vi "close camera.vi"(8 "error in (no error)":errorcluster, 11 "Camera":T1) -> (0 "error out":errorcluster, 3 "Camera out":T1)   [LabVIEW 2022 SP3, in "Vision.lvlib"]
uses:
  Vision.lvlib
  camera.ctl
  camera driver.ctl
  C:/Users/Caleb/Desktop/nebraska-silicon-lab/pixel-gantry-extra/LV/bin/uEyeDotNet.dll
  bin/uEyeDotNet.dll
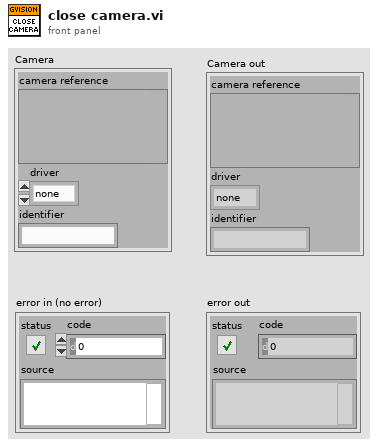
[diagram p1: front panel]
types:
  T1 = typedef "Vision.lvlib/camera.ctl" = cluster{"camera reference":variant, "driver":T2, "identifier":string}
  T2 = typedef "Vision.lvlib/camera driver.ctl" = enum16{"none", "ueye", "wmf"}
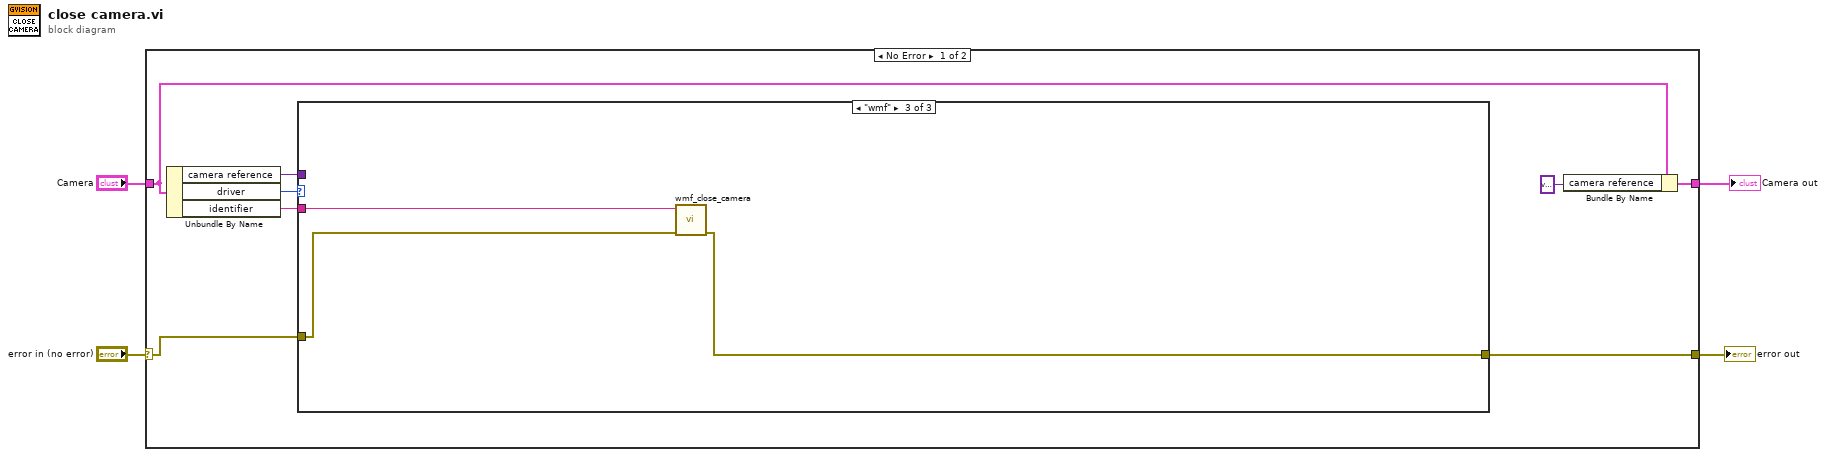
[diagram p0: block diagram]
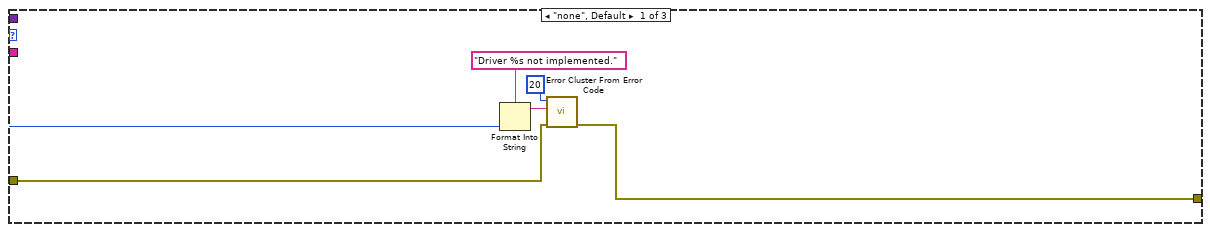
[diagram p2: hidden frame]
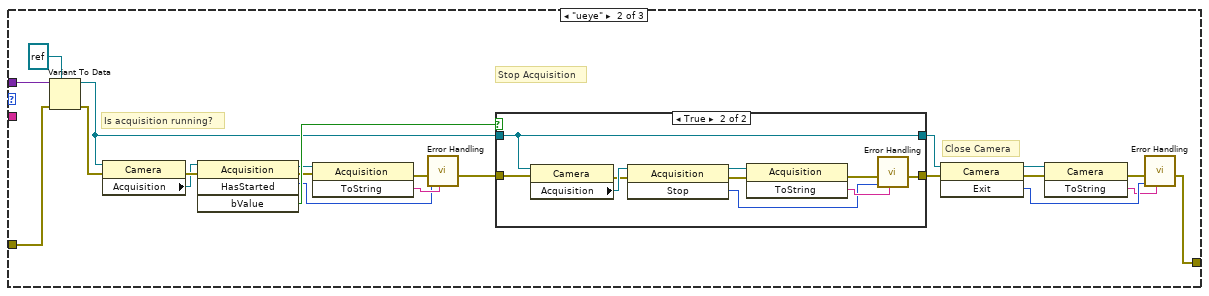
[diagram p3: hidden frame]
diagram:
  n1 = case shown="No Error" "error in (no error)" {
    selector: "error in (no error)" -> [w12 w57]
    tunnel: [w9 w57] -> w3
    tunnel: "Camera" -> [w8 w56]
    tunnel: [w6 w56] -> w1
    frame No Error {
      n2 = Unbundle By Name(w8) -> ("camera reference"=w10:variant, "driver"=w11:T2, "identifier"=w5:string)
      n3 = case shown="\"wmf\"" w11 {
        selector: w11 -> [w15 _ _]
        tunnel: w12 -> [w17 w29 w54]
        tunnel: w10 -> [_ w39 _]
        tunnel: [w13 w19 w53] -> w9
        tunnel: w5 -> [_ _ w55]
        frame "none", Default {
          n4 = Format Into String(format string="Driver %s not implemented.", w15) -> (resulting string=w14:string)  [unwired: 2 in, 1 out]
          n5 = call <vilib>:"Error Cluster From Error Code.vi"("error in (no error)"=w17, "error message (\"\")"=w14, "error code (0)"=20) -> ("error out"=w13:errorcluster)  [unwired: 6 in]
        }
        frame "ueye" {
          # "Close Camera"
          # "Is acquisition running?"
          # "Stop Acquisition"
          n6 = Variant To Data(error in=w29, type=refnum<k24> refnum ("reference"), Variant=w39) -> (data=w27:refnum<k24>, error out=w28:errorcluster)
          n7 = property class="Camera"(reference=w27, error in=w28) -> (error out=w38:errorcluster, "Acquisition"=w37:refnum<k24>)  [unwired: 1 out]
          n8 = invoke class="Acquisition" method="HasStarted"(reference=w37, error in=w38) -> (reference out=w34:refnum<k24>, error out=w35:errorcluster, "HasStarted"=w31:i32, "bValue"=w36:bool)  [unwired: 2 in]
          n9 = invoke class="Acquisition" method="ToString"(reference=w34, error in=w35) -> (error out=w33:errorcluster, "ToString"=w32:string)  [unwired: 1 in, 1 out]
          n10 = call "Error Handling.vi"("Error String"=w32, "Error Code"=w31, "Error In"=w33) -> ("Error Out"=w30:errorcluster)  [unwired: 8 in]
          n11 = case shown="True" w36 {
            tunnel: [w42 w43] -> w23
            tunnel: w30 -> [w42 w52]
            tunnel: w27 -> [w41 w47]
            tunnel: [w41 w47] -> w24
            frame False {
            }
            frame True {
              n12 = property class="Camera"(reference=w47, error in=w52) -> (error out=w50:errorcluster, "Acquisition"=w51:refnum<k24>)  [unwired: 1 out]
              n13 = invoke class="Acquisition" method="Stop"(reference=w51, error in=w50) -> (reference out=w48:refnum<k24>, error out=w49:errorcluster, "Stop"=w44:i32)  [unwired: 1 in]
              n14 = invoke class="Acquisition" method="ToString"(reference=w48, error in=w49) -> (error out=w46:errorcluster, "ToString"=w45:string)  [unwired: 1 in, 1 out]
              n15 = call "Error Handling.vi"("Error String"=w45, "Error Code"=w44, "Error In"=w46) -> ("Error Out"=w43:errorcluster)  [unwired: 8 in]
            }
          }
          n16 = invoke class="Camera" method="Exit"(reference=w24, error in=w23) -> (reference out=w25:refnum<k24>, error out=w26:errorcluster, "Exit"=w21:i32)  [unwired: 1 in]
          n17 = invoke class="Camera" method="ToString"(reference=w25, error in=w26) -> (error out=w22:errorcluster, "ToString"=w20:string)  [unwired: 1 in, 1 out]
          n18 = call "Error Handling.vi"("Error String"=w20, "Error Code"=w21, "Error In"=w22) -> ("Error Out"=w19:errorcluster)  [unwired: 8 in]
        }
        frame "wmf" {
          n19 = call "wmf_close_camera.vi"("error in (no error)"=w54, "camera_name"=w55) -> ("error out"=w53:errorcluster)  [unwired: 9 in]
        }
      }
      n20 = Bundle By Name(cluster=w8, "camera reference"=variant) -> (w6:T1)
    }
    frame Error {
    }
  }
  "error out" <- w3
  "Camera out" <- w1
